vi "Pressure reg code.vi"() -> ()   [LabVIEW 2016]
uses:
  <vilib>/Utility/file.llb/Write Delimited Spreadsheet (DBL).vi
  <vilib>/measure/NI_MABase.lvlib
  <vilib>/ptbypt/NI_PtbyPt.lvlib
panel:
  out "Array":dbl[](array[numeric])
  out "Waveform Chart 2":dbl(graph)
  out "Waveform Chart":dynamicdata(graph)
  in  "data 3":dbl(slide) scale=0.0..0.02
  out "data 2":dbl
  out "sin(x)":dbl
  out "x-y*floor(x/y)":i32
  out "Y":dbl[](array[numeric])
  in  "stop":bool
  in  "data":dbl
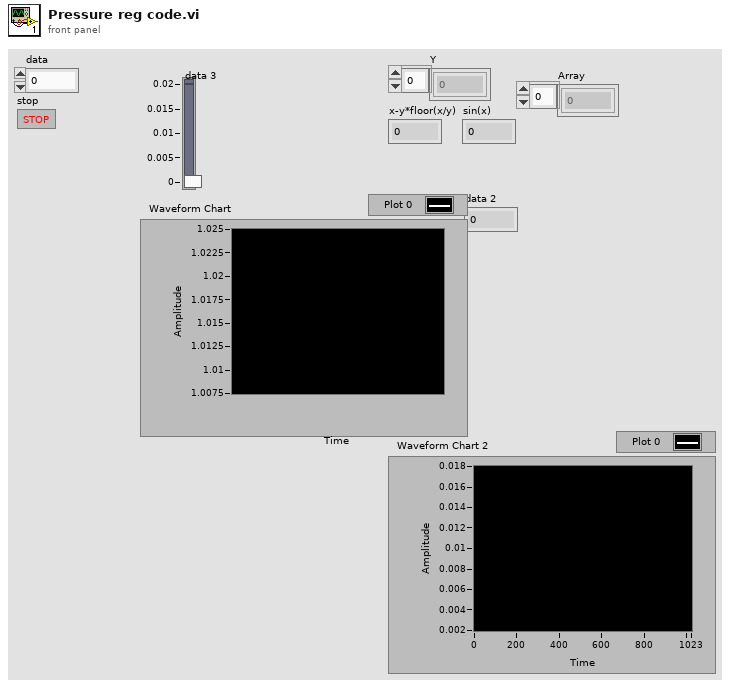
[diagram p1: front panel]
types:
  T1 = enum16{"Sine Wave", "Triangle Wave", "Square Wave", "Sawtooth Wave"}
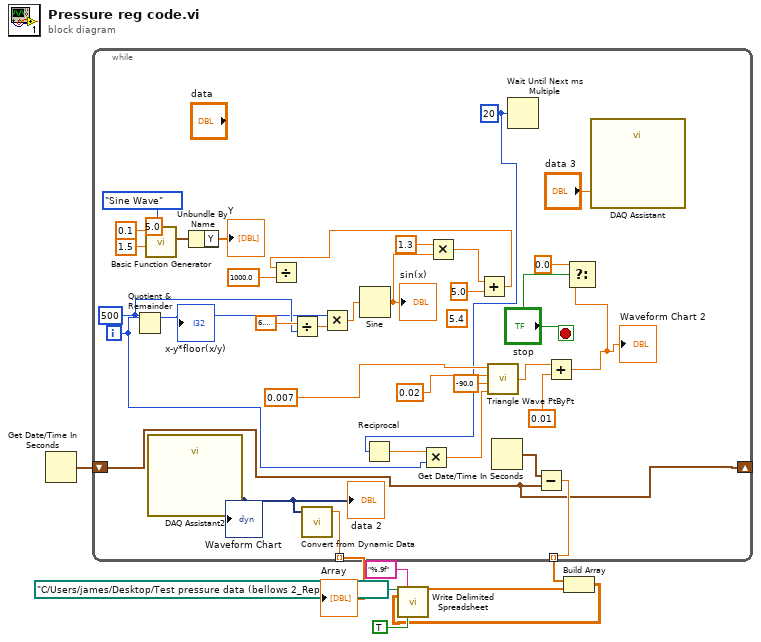
[diagram p0: block diagram]
diagram:
  n1 = Get Date/Time In Seconds() -> (seconds since 1Jan1904=w4:timestamp)
  n2 = while {
    tunnel: [w13] -> w2 mode=indexing
    shift-right: [w10] -> _
    shift-left: w4 -> [w10]
    tunnel: [w11] -> w3 mode=indexing
    i -> [w18]
    stop <- "stop" stop-if-true
    (unwired) 5.4 ("y")
    w34 = 500 ("x")
    w20 = u32 20 ("millisecond multiple")
    n3 = Quotient & Remainder(x=w18, y=w34) -> (x-y*floor(x/y)=w32:i32)  [unwired: 1 out]
    "x-y*floor(x/y)" <- w32
    n4 = call <vilib>:"Basic Function Generator.vi"("offset"=5.0, "signal type"=T1."Sine Wave", "amplitude"=1.5, "frequency"=0.1) -> ("signal out"=w37:waveform(dbl))  [unwired: 5 in, 2 out]
    n5 = call "DAQ Assistant2"() -> ("data"=w14:dynamicdata)  [unwired: 17 in, 2 out]
    "data 2" <- w14
    "Waveform Chart" <- w14
    n6 = Unbundle By Name(w37) -> ("Y"=→"Y":dbl[])
    n7 = Divide(x=6.283185307179586, y=w34) -> (x/y=w33:dbl)
    n8 = call "Convert from Dynamic Data"("Dynamic Data Type"=w14) -> ("Scalar"=w13:dbl)  [unwired: 3 in]
    n9 = Multiply(x=w32, y=w33) -> (x*y=w31:dbl)
    n10 = Sine(x=w31) -> (sin(x)=w29:dbl)
    "sin(x)" <- w29
    n11 = Reciprocal(x=w20) -> (1/x=w19:dbl)
    n12 = Multiply(x=w19, y=w18) -> (x*y=w17:dbl)
    n13 = Multiply(x=1.3, y=w29) -> (x*y=w27:dbl)
    n14 = Add(x=w27, y=5.0) -> (x+y=w26:dbl)
    n15 = Divide(x=w26, y=1000.0) -> ()  [unwired: 1 out]
    n16 = call <vilib>:"Triangle Wave PtByPt.vi"("time"=w17, "phase"=-90.0, "frequency"=0.02, "amplitude"=0.007) -> ("triangle wave"=w22:dbl)
    n17 = Get Date/Time In Seconds() -> (seconds since 1Jan1904=w12:timestamp)
    n18 = Wait Until Next ms Multiple(millisecond multiple=w20) -> ()  [unwired: 1 out]
    n19 = Subtract(x=w12, y=w10) -> (x-y=w11:dbl)
    n20 = Add(x=w22, y=0.01 ("offset")) -> (x+y=w15:dbl)
    "Waveform Chart 2" <- w15
    n21 = Select(t=0.0, s="stop", f=w15) -> ()  [unwired: 1 out]
    n22 = call "DAQ Assistant"("data"="data 3") -> ()  [unwired: 17 in, 2 out]
  }
  "Array" <- w2
  n23 = Build Array(w3, w2) -> (w1:dbl[][])
  n24 = call-poly <vilib>:"Write Delimited Spreadsheet.vi"("file path (dialog if empty)"=path "C:/Users/james/Desktop/Test pressure data (bellows 2_Rep_5).txt", "format (%.3f)"="%.9f", "2D data"=w1, "transpose? (no:F)"=TRUE) -> ()  [unwired: 10 in, 2 out]
